vi "Log_Foco.vi"(6 "command":string, 7 "focValue":string, 8 "pathLogFocoString":string) -> ()   [LabVIEW 2012]
panel:
  out "Date":string
  in  "pathLogFoco":path
  out "error out":errorcluster
  out "writingLog":bool
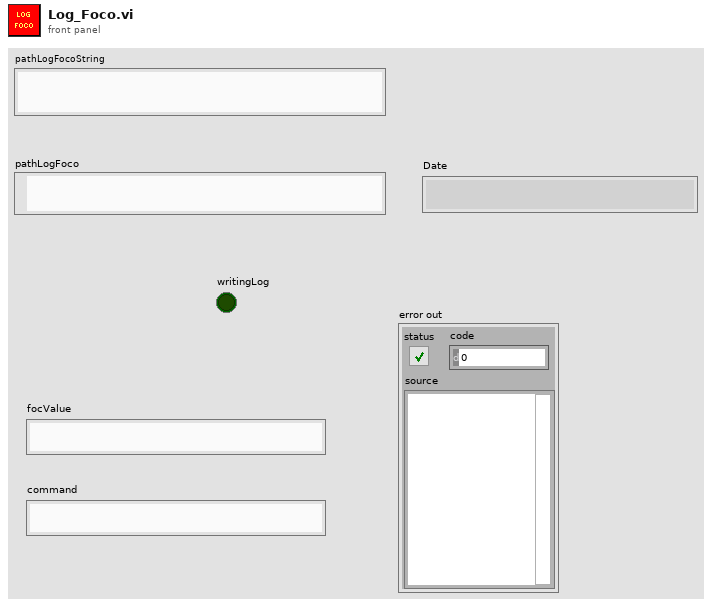
[diagram p1: front panel]
types:
  T1 = enum16{"open", "replace", "create", "open or create", "replace or create", "replace or create with confirmation"}
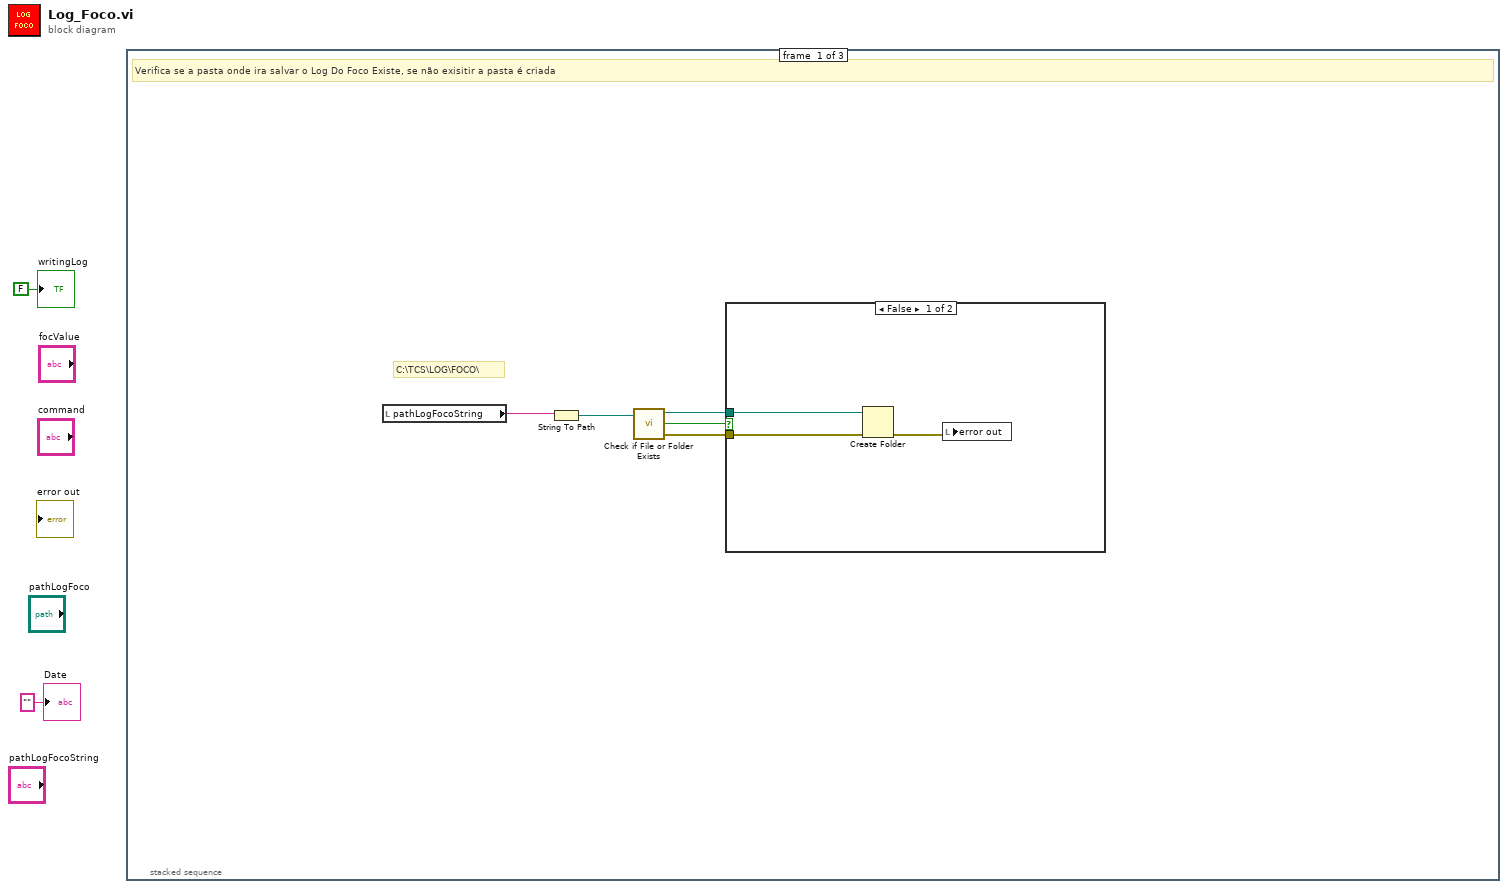
[diagram p0: block diagram]
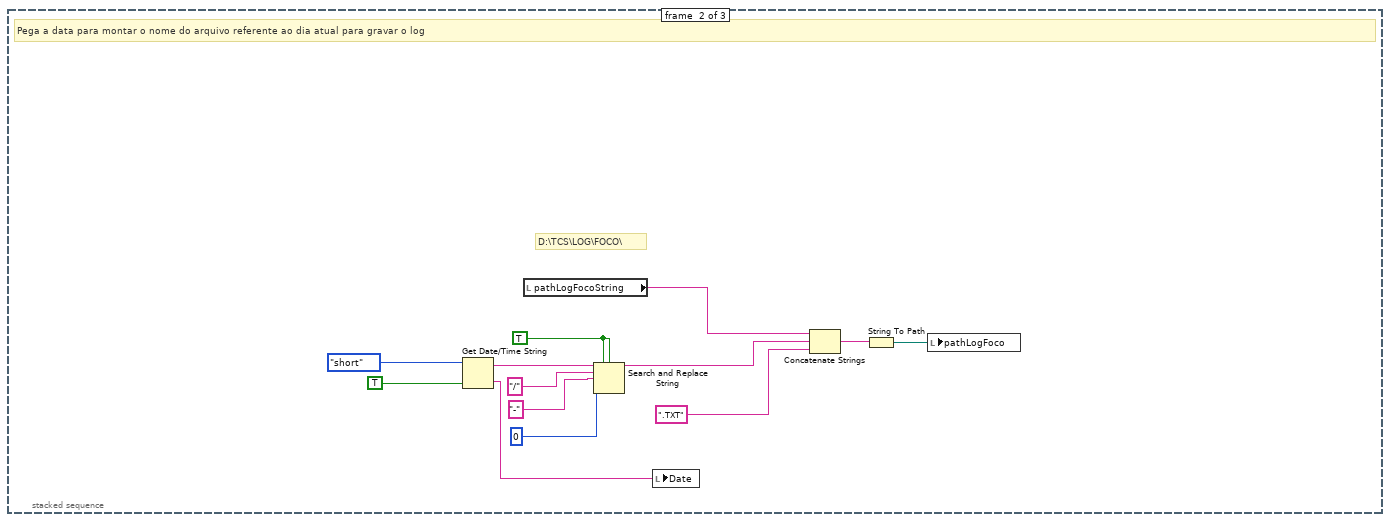
[diagram p3: hidden frame]
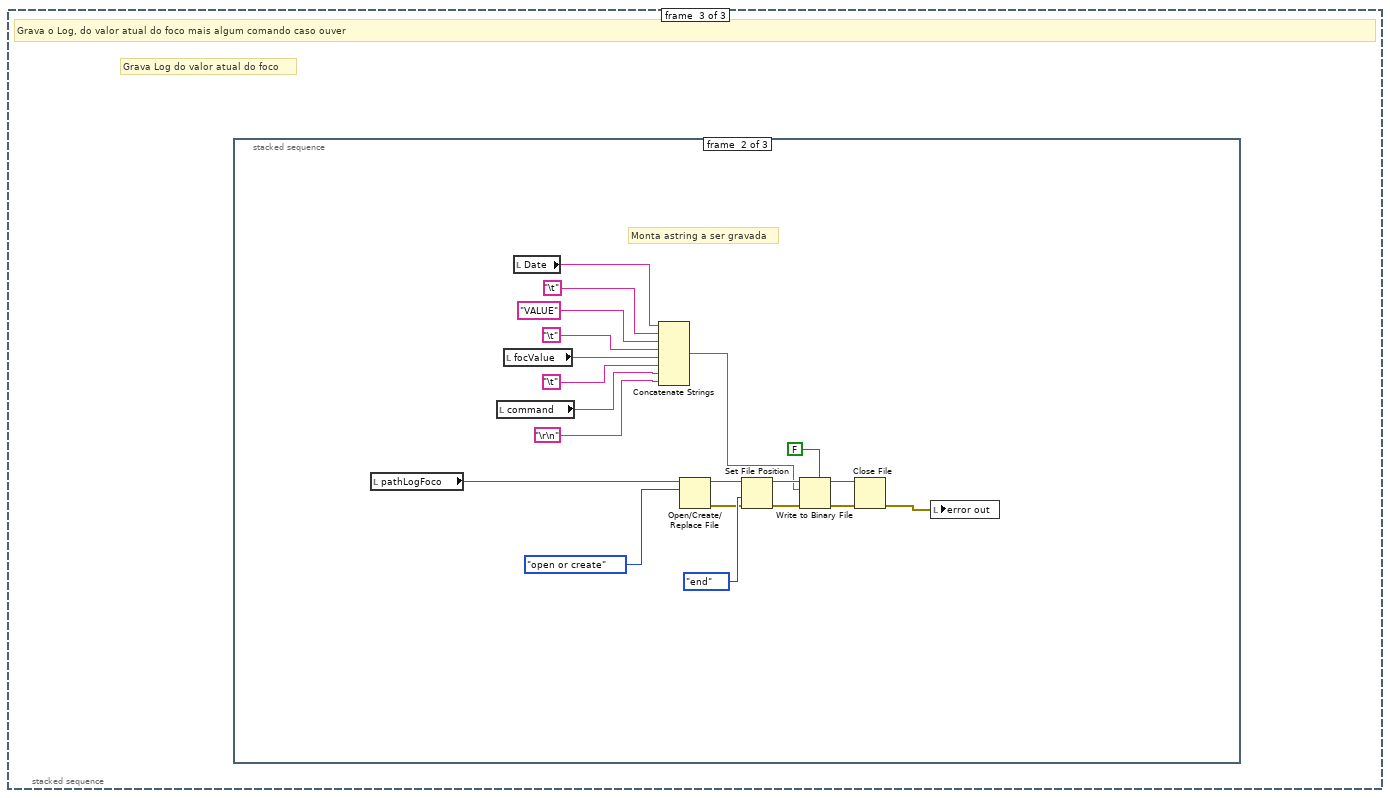
[diagram p4: hidden frame]
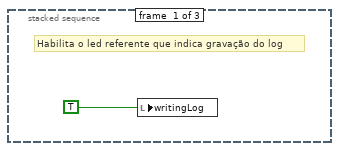
[diagram p5: hidden frame]
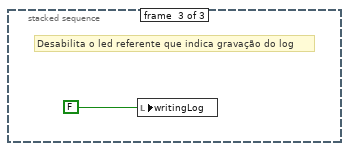
[diagram p6: hidden frame]
diagram:
  n1 = stacked-sequence {
    frame #0 {
      # "C:\\TCS\\LOG\\FOCO\\"
      # "Verifica se a pasta onde ira salvar o Log Do Foco Existe, se não exisitir a pasta é criada"
      n2 = local read "pathLogFocoString"() -> (w4:string)
      n3 = String To Path(string=w4) -> (path=w3:path)
      n4 = call <vilib>:"Check if File or Folder Exists.vi"("path"=w3) -> ("error out"=w5:errorcluster, "file or folder exists?"=w7:bool, "dup path"=w6:path)  [unwired: 8 in]
      n5 = case shown="False" w7 {
        tunnel: w6 -> [w10 _]
        tunnel: w5 -> [w9 _]
        frame False {
          n6 = Create Folder(path (use dialog)=w10, error in=w9) -> (error out=w8:errorcluster)  [unwired: 1 in, 2 out]
          n7 = local write "error out"(w8) -> ()
        }
        frame True {
        }
      }
    }
    frame #1 {
      w15 = TRUE ("replace all? (F)")
      # "D:\\TCS\\LOG\\FOCO\\"
      # "Pega a data para montar o nome do arquivo referente ao dia atual para gravar o log"
      n8 = Get Date/Time String(date format (0)=enum16{"short", "long", "abbreviated"}."short", want seconds? (F)=TRUE) -> (date string=w19:string, time string=w12:string)  [unwired: 1 in]
      n9 = local read "pathLogFocoString"() -> (w11:string)
      n10 = Search and Replace String(replace all?=w15, case sensitive?=w15, input string=w19, search string="/" ("replace string (\"\")"), replace string="-" ("replace string (\"\")"), offset=0 ("offset (0)")) -> (result string=w13:string)  [unwired: 2 in, 3 out]
      n11 = local write "Date"(w12) -> ()
      n12 = Concatenate Strings(w11, w13, ".TXT" ("SOMENTE DIRETORIO")) -> (w22:string)
      n13 = String To Path(string=w22) -> (path=w14:path)
      n14 = local write "pathLogFoco"(w14) -> ()
    }
    frame #2 {
      # "Grava Log do valor atual do foco"
      # "Grava o Log, do valor atual do foco mais algum comando caso ouver"
      n15 = stacked-sequence {
        frame #0 {
          # "Habilita o led referente que indica gravação do log"
          n16 = local write "writingLog"(TRUE) -> ()
        }
        frame #1 {
          # "Monta astring a ser gravada"
          n17 = local read "pathLogFoco"() -> (w44:path)
          n18 = local read "command"() -> (w26:string)
          n19 = local read "focValue"() -> (w33:string)
          n20 = local read "Date"() -> (w29:string)
          n21 = Concatenate Strings(w29, "\t", "VALUE", "\t", w33, "\t", w26, "\r\n") -> (w32:string)
          n22 = Open/Create/Replace File(file path (use dialog)=w44, operation (0:open)=T1."open or create") -> (refnum out=w42:refnum<file>, error out=w38:errorcluster)  [unwired: 4 in, 1 out]
          n23 = Set File Position(refnum=w42, from (0:start)=enum16{"start", "end", "current"}."end", error in=w38) -> (refnum out=w39:refnum<file>, error out=w40:errorcluster)  [unwired: 1 in]
          n24 = Write to Binary File(file (use dialog)=w39, data=w32, error in=w40, 5:FALSE ("prepend array or string size? (T)")) -> (refnum out=w36:refnum<file>, error out=w35:errorcluster)  [unwired: 2 in, 1 out]
          n25 = Close File(refnum=w36, error in=w35) -> (error out=w34:errorcluster)  [unwired: 1 out]
          n26 = local write "error out"(w34) -> ()
        }
        frame #2 {
          # "Desabilita o led referente que indica gravação do log"
          n27 = local write "writingLog"(FALSE) -> ()
        }
      }
    }
  }
  "writingLog" <- FALSE ("writingLog")
  "Date" <- "" ("Date")
